vi "heart rate monitor simulation.vi"() -> ()   [LabVIEW 2019]
uses:
  <vilib>/sound2/lvsound2.llb/Sound File Read Open.vi
  <vilib>/sound2/lvsound2.llb/Sound File Read (DBL).vi
  <vilib>/measure/mamon.llb/Waveform Peak Detection for N Chan.vi
  <vilib>/measure/NI_MAPro.lvlib
panel:
  in  "stop 2":bool
  out "error out":errorcluster
  in  "error in (no error)":errorcluster
  out "Waveform Chart":dynamicdata(graph)
  out "Waveform Graph":dynamicdata(graph)
  in  "stop":bool
  out "Heart Rate":dbl
  out "Frequency in Hz":dbl
  out "Scalar":dbl
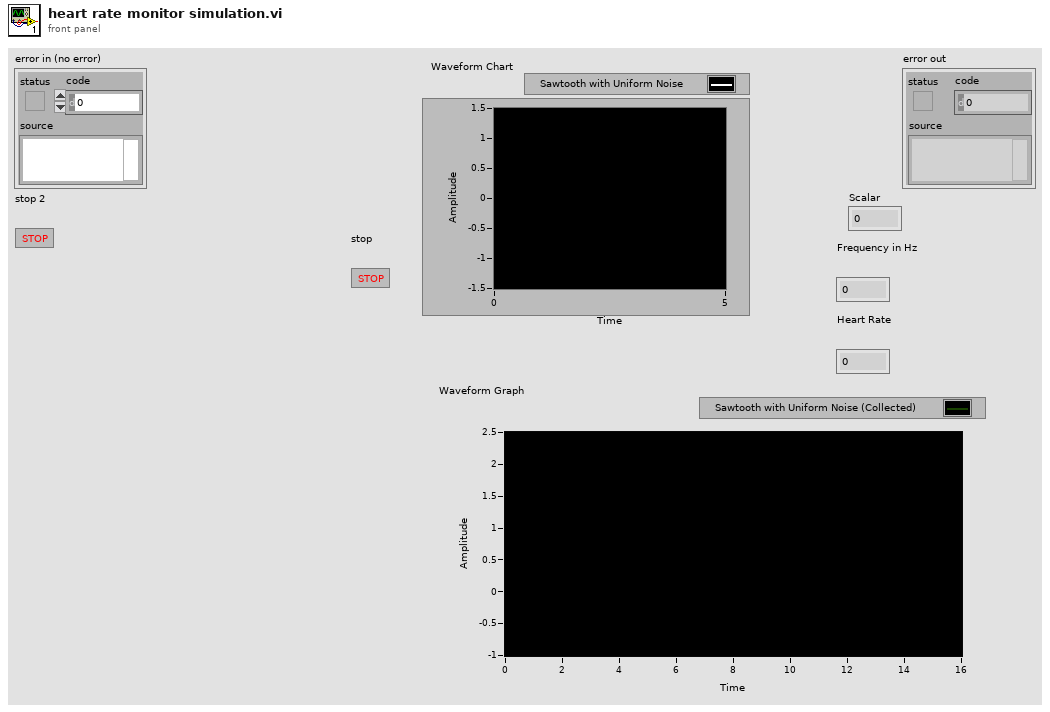
[diagram p1: front panel]
types:
  T1 = typedef "Sound File Refnum.ctl" = refnum<file>
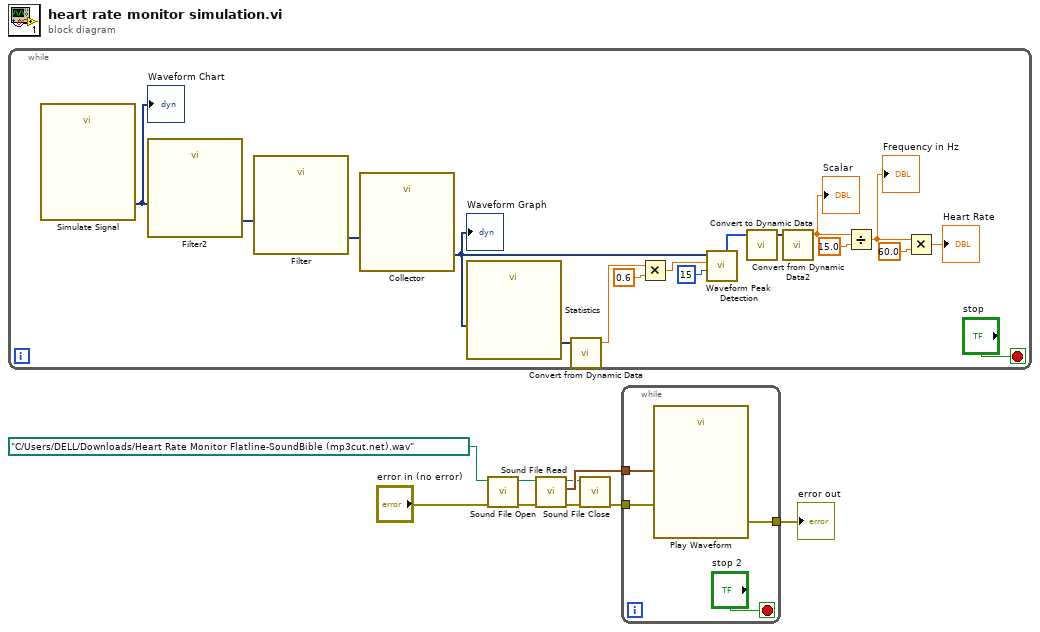
[diagram p0: block diagram]
diagram:
  n1 = while {
    stop <- "stop" stop-if-true
    n2 = call "Simulate Signal"() -> ("Sawtooth with Uniform Noise"=w13:dynamicdata)  [unwired: 14 in, 1 out]
    "Waveform Chart" <- w13
    n3 = call "Filter2"("Signal"=w13) -> ("Filtered Signal"=w26:dynamicdata)  [unwired: 9 in, 1 out]
    n4 = call "Filter"("Signal"=w26) -> ("Filtered Signal"=w15:dynamicdata)  [unwired: 9 in, 1 out]
    n5 = call "Collector"("Signals"=w15) -> ("Collected Signals"=w14:dynamicdata)  [unwired: 9 in, 1 out]
    "Waveform Graph" <- w14
    n6 = call "Statistics"("Signals"=w14) -> ("Maximum"=w25:dynamicdata)  [unwired: 25 in, 1 out]
    n7 = call "Convert from Dynamic Data"("Dynamic Data Type"=w25) -> ("Scalar"=w24:dbl)  [unwired: 3 in]
    n8 = Multiply(x=w24, y=0.6) -> (x*y=w21:dbl)
    n9 = call-poly <vilib>:"Waveform Peak Detection.vi"("width"=15, "threshold"=w21, "Signals In"=w14) -> ("# found"=w19:i32[])  [unwired: 4 in, 4 out]
    n10 = call "Convert to Dynamic Data"("Array"=w19) -> ("Dynamic Data Type"=w20:dynamicdata)  [unwired: 3 in]
    n11 = call "Convert from Dynamic Data2"("Dynamic Data Type"=w20) -> ("Scalar"=w11:dbl)  [unwired: 3 in]
    "Scalar" <- w11
    n12 = Divide(x=w11, y=15.0) -> (x/y=w10:dbl)
    "Frequency in Hz" <- w10
    n13 = Multiply(x=w10, y=60.0) -> (x*y=→"Heart Rate":dbl)
  }
  n14 = call-poly <vilib>:"Sound File Open.vi"("error in (no error)"="error in (no error)", "path"=path "C:/Users/DELL/Downloads/Heart Rate Monitor Flatline-SoundBible (mp3cut.net).wav") -> ("error out"=w5:errorcluster, "sound file refnum"=w8:T1)  [unwired: 8 in]
  n15 = call-poly <vilib>:"Sound File Read.vi"("error in (no error)"=w5, "sound file refnum"=w8) -> ("error out"=w6:errorcluster, "data"=w7:waveform(dbl)[], "sound file refnum out"=w2:T1)  [unwired: 5 in, 2 out]
  n16 = call <vilib>:"Sound File Close.vi"("error in (no error)"=w6, "sound file refnum"=w2) -> ("error out"=w3:errorcluster)  [unwired: 9 in]
  n17 = while {
    tunnel: w7 -> [w30]
    tunnel: w3 -> [w29]
    tunnel: [w28] -> w1
    stop <- "stop 2" stop-if-true
    n18 = call "Play Waveform"("Data"=w30, "error in"=w29) -> ("error out"=w28:errorcluster)  [unwired: 17 in]
  }
  "error out" <- w1
